vi "SimpleNumbertoString.vi"(1 "Numeric":i32) -> (0 "String":string)   [LabVIEW 2010]
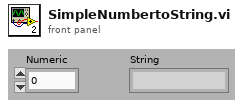
[diagram p1: front panel]
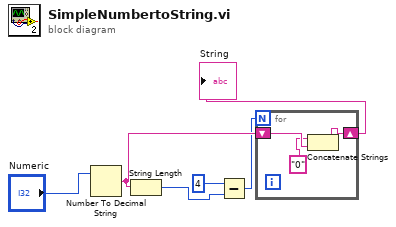
[diagram p0: block diagram]
diagram:
  n1 = Number To Decimal String(number="Numeric") -> (decimal integer string=w5:string)  [unwired: 1 in]
  n2 = String Length(string=w5) -> (length=w3:i32)
  n3 = Subtract(x=4, y=w3) -> (x-y=w4:i32)
  n4 = for {
    N: w4 -> [_]
    shift-right: [w7] -> w6
    shift-left: w5 -> [w9]
    n5 = Concatenate Strings("0", w9) -> (w7:string)
  }
  "String" <- w6
